vi "Layer Write Low Level.vi"(8 "error in (no error)":errorcluster, 9 "Batch ID":i32, 10 "Layer Information Cluster":T1 {"Deposition Method" items=["Front Electrode", "Electron Transport Layer", "Active Layer", "Hole Transport Layer", "Back Electrode", "Custom Layer"]; "Layer Type" items=["Front Electrode", "Electron Transport Layer", "Active Layer", "Hole Transport Layer", "Back Electrode", "Custom Layer"]}, 11 "Database Connection In":T2) -> (0 "error out":errorcluster, 3 "Database Connection Out":T2)   [LabVIEW 2020]
uses:
  <vilib>/addons/database/Connection.llb/Conn ObjectReference.ctl
  Data Clusters/Layer Information Cluster.ctl
  <vilib>/addons/database/NI_Database_API.lvlib
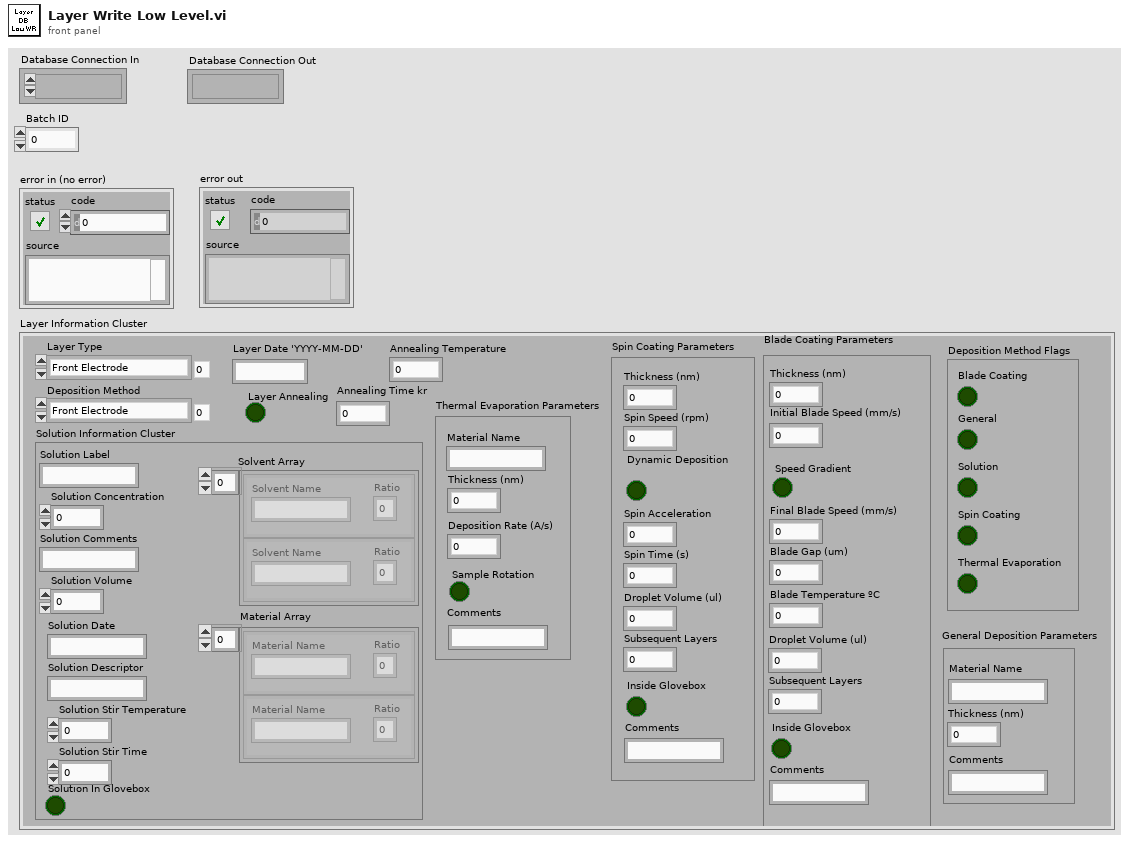
[diagram p1: front panel]
types:
  T1 = typedef "Layer Information Cluster.ctl" = cluster{"Solution Information Cluster":cluster{"Solution Label":string, "Solution Concentration":dbl, "Solution Comments ":string, "Solution Volume ":dbl, "Solution Date ":string, "Solution Descriptor ":string, "Solution Stir Temperature ":dbl, "Solution Stir Time ":dbl, "Solution In Glovebox":bool, "Solvent Array":cluster{"Solvent Name":string, "Ratio":dbl}[], "Material Array":cluster{"Material Name":string, "Ratio":dbl}[]}, "Layer Type":u16, "Deposition Method":u16, "Layer Annealing":bool, "General Deposition Parameters":cluster{"Thickness (nm)":dbl, "Comments":string, "Material Name":string}, "Blade Coating Parameters":cluster{"Thickness (nm)":dbl, "Initial Blade Speed (mm/s)":dbl, "Speed Gradient":bool, "Final Blade Speed (mm/s)":dbl, "Blade Gap (um)":dbl, "Droplet Volume (ul)":dbl, "Subsequent Layers":dbl, "Inside Glovebox":bool, "Comments":string, "Blade Temperature ºC":dbl}, "Spin Coating Parameters":cluster{"Thickness (nm)":dbl, "Spin Speed (rpm)":dbl, "Dynamic Deposition":bool, "Spin Acceleration":dbl, "Spin Time (s)":dbl, "Droplet Volume (ul)":dbl, "Subsequent Layers":dbl, "Inside Glovebox":bool, "Comments":string}, "Thermal Evaporation Parameters":cluster{"Deposition Rate (A/s)":dbl, "Thickness (nm)":dbl, "Comments":string, "Material Name":string, "Sample Rotation":bool}, "Layer Date 'YYYY-MM-DD'":string, "Annealing Time kr":dbl, "Annealing Temperature":dbl, "Deposition Method Flags":cluster{"Blade Coating":bool, "General ":bool, "Solution":bool, "Spin Coating":bool, "Thermal Evaporation":bool}}
  T2 = typedef "NI_Database_API.lvlib/Conn ObjectReference.ctl" = refnum<k1>
  T3 = cluster{"Layer Type":u16, "Deposition Method":u16, "Layer Annealing":bool, "Annealing Temperature":dbl, "Annealing Time kr":dbl, "Layer Date ":string, "Batch ID":i32}
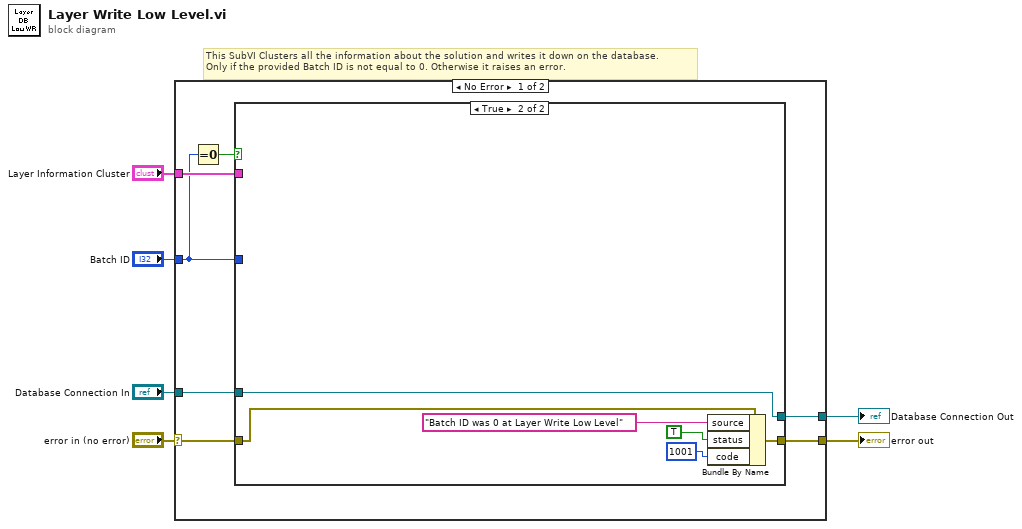
[diagram p0: block diagram]
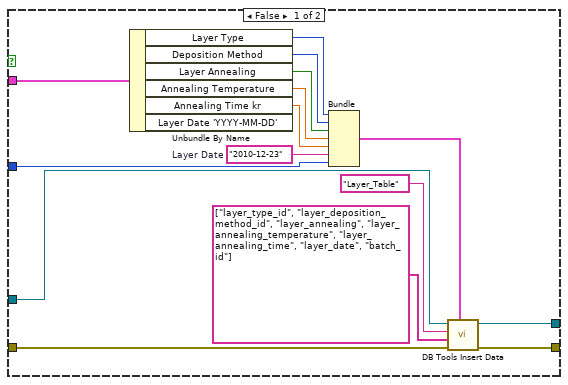
[diagram p2: hidden frame]
diagram:
  # "This SubVI Clusters all the information about the solution and writes it down on the database.\nOnly if the provided Batch ID is not equal to 0. Otherwise it raises an error."
  n1 = case shown="No Error" "error in (no error)" {
    selector: "error in (no error)" -> [w10 w35]
    tunnel: [w13 w35] -> w6
    tunnel: [w12 w36] -> w5
    tunnel: "Database Connection In" -> [w11 w36]
    tunnel: "Layer Information Cluster" -> [w9 _]
    tunnel: "Batch ID" -> [w8 _]
    frame No Error {
      n2 = Equal To 0?(x=w8) -> (x = 0?=w7:bool)
      n3 = case shown="True" w7 {
        tunnel: [w28 w31] -> w13
        tunnel: [w27 w34] -> w12
        tunnel: w11 -> [w26 w34]
        tunnel: w10 -> [w25 w33]
        tunnel: w9 -> [w23 _]
        tunnel: w8 -> [w14 _]
        frame False {
          w17 = "2010-12-23"  # Layer Date
          n4 = Unbundle By Name(w23) -> ("Layer Type"=w22:u16, "Deposition Method"=w21:u16, "Layer Annealing"=w20:bool, "Annealing Temperature"=w19:dbl, "Annealing Time kr"=w18:dbl)  [unwired: 1 out]
          n5 = Bundle("Layer Type"=w22, "Deposition Method"=w21, "Layer Annealing"=w20, "Annealing Temperature"=w19, "Annealing Time kr"=w18, "Layer Date"=w17, "Batch ID"=w14) -> (w16:T3)  [unwired: 1 in]
          n6 = call <vilib>:"DB Tools Insert Data.vi"("data"=w16, "error in (no error)"=w25, "columns"=string[] ["layer_type_id", "layer_deposition_method_id", "layer_annealing", "layer_annealing_temperature", "layer_annealing_time", "layer_date", "batch_id"], "table"="Layer_Table", "connection reference"=w26) -> ("error out"=w28:errorcluster, "connection reference out"=w27:T2)  [unwired: 5 in]
        }
        frame True {
          n7 = Bundle By Name(cluster=w33, "source"="Batch ID was 0 at Layer Write Low Level", "status"=TRUE, "code"=1001) -> (w31:errorcluster)
        }
      }
    }
    frame Error {
    }
  }
  "error out" <- w6
  "Database Connection Out" <- w5
